vi "Task 1 CFU.vi"() -> ()   [LabVIEW 2016]
panel:
  out "String 2":string
  in  "pH":dbl
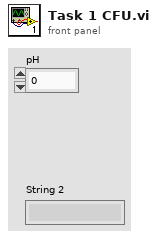
[diagram p1: front panel]
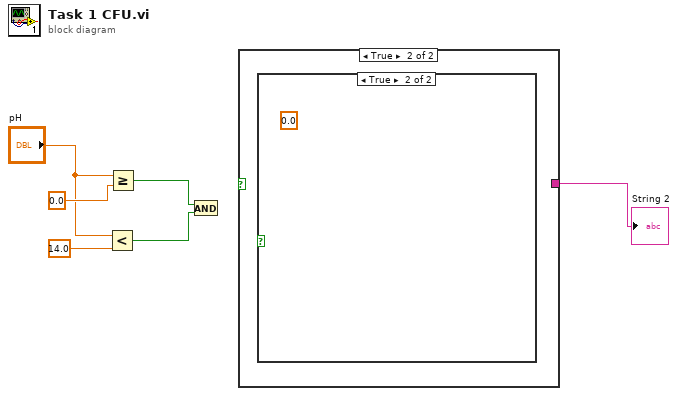
[diagram p0: block diagram]
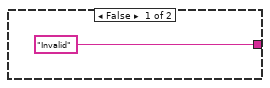
[diagram p2: hidden frame]
diagram:
  n1 = Less?(x="pH", y=14.0) -> (x < y?=w3:bool)
  n2 = Greater Or Equal?(x="pH", y=0.0) -> (x >= y?=w2:bool)
  n3 = And(x=w2, y=w3) -> ()  [unwired: 1 out]
  n4 = case shown="True" {
    selector: _ -> [_ _]
    tunnel: ["Invalid" _] -> w1
    frame False {
    }
    frame True {
      n5 = case shown="True" {
        selector: _ -> [_ _]
        frame False {
        }
        frame True {
          (unwired) 0.0
        }
      }
    }
  }
  "String 2" <- w1
